vi "testErrorPassesThrough.vi"() -> ()   [LabVIEW 2017, in "Transparent Assertions.Tests.lvlib" / "ExpectationFailedError.lvlib"]
uses:
  ExpectationFailedError.lvlib
  <vilib>/Utility/error.llb/Error Cluster From Error Code.vi
  <vilib>/ErrorRing/Error Ring.xnode
  src/Transparent Assertions/Transparent Assertions.lvlib
panel:
  out "error out":errorcluster
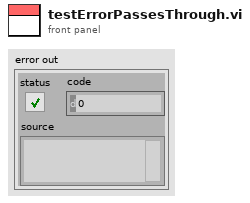
[diagram p1: front panel]
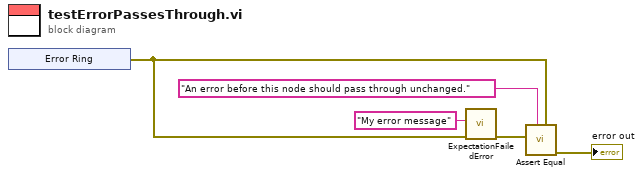
[diagram p0: block diagram]
diagram:
  n1 = xnode "Error Ring"() -> ("error out"=w2:errorcluster)
  n2 = call "ExpectationFailedError.vi"("error in (no error)"=w2, "Message"="My error message") -> ("error out"=w4:errorcluster)  [unwired: 9 in]
  n3 = call "Assert Equal.vi"("Expected"=w2, "Message (\"\")"="An error before this node should pass through unchanged." ("Message (\"\")"), "Actual"=w4) -> ("error out"=→"error out":errorcluster)  [unwired: 8 in]
